vi "crio_9074_FPGA_Load_Cell_new.vi"() -> ()   [LabVIEW 2019]
uses:
  <vilib>/LabVIEW Targets/FPGA/cRIO/shared/nicrio_ModuleControls/nicrio_cRIO-9237_DataRatesRing.ctl
  <vilib>/LabVIEW Targets/FPGA/cRIO/shared/nicrio_ModuleControls/nicrio_cRIO-9237_ExcitationVoltageRing.ctl
  <vilib>/rvi/Emulation/niFpgaSctlEmulationGetInTimedLoop.vi
  <vilib>/rvi/Emulation/niFpgaProcessEmulError.vi
  <vilib>/rvi/eio/common/nirviEmuTemplatePropertySet_errors.vi
  <vilib>/rvi/eio/common/nirviEmuTemplateMethod_errors.vi
  <vilib>/rvi/Emulation/niFpgaGetClockAttributes.vi
  <vilib>/rvi/Emulation/niFpgaEmulationReportErrorSimple.vi
  <vilib>/rvi/Emulation/niFpgaCriticalErrorInLSC.vi
  <vilib>/eio/EIOPropertyNode/EIOPropertyNode.xnode
  <vilib>/eio/EIONode/EIONode.xnode
  <vilib>/rvi/eio/common/nirviEmuTemplatePropertyGet_errors.vi
  <vilib>/rvi/eio/common/nirviEmuTemplatePropertyGet_noerrors.vi
  <vilib>/rvi/eio/common/nirviEmuTemplatePropertySet_noerrors.vi
panel:
  in  "Loop Rate (uSec)":u32
  out "Mod1/AI0":fxp<+/-,24,-4>
  in  "Half-Bridge Enable":bool
  in  "Excitation Voltage":T1 items=["2.5 Volts", "3.3 Volts", "5.0 Volts", "10.0 Volts", "External Excitation"]
  in  "Finite?":bool=TRUE
  in  "Samples per Channel":u32=1000
  in  "Shunt Cal Enable":bool
  in  "Stop Button":bool
  in  "Data Rate":T2=1 items=["50.000 kS/s (NI 9237)"=1, "25.000 kS/s (NI 9237)"=2, "16.667 kS/s (NI 9237)"=3, "12.500 kS/s (NI 9237)"=4, "10.000 kS/s (NI 9237)"=5, "8.333 kS/s (NI 9237)"=6, "7.143 kS/s (NI 9237)"=7, "6.250 kS/s (NI 9237)"=8, "5.556 kS/s (NI 9237)"=9, "5.000 kS/s (NI 9237)"=10, "4.545 kS/s (NI 9237)"=11, "4.167 kS/s (NI 9237)"=12, "3.846 kS/s (NI 9237)"=13, "3.571 kS/s (NI 9237)"=14, "3.333 kS/s (NI 9237)"=15, "3.125 kS/s (NI 9237)"=16, "2.941 kS/s (NI 9237)"=17, "2.778 kS/s (NI 9237)"=18, "2.632 kS/s (NI 9237)"=19, "2.500 kS/s (NI 9237)"=20, "2.381 kS/s (NI 9237)"=21, "2.273 kS/s (NI 9237)"=22, "2.174 kS/s (NI 9237)"=23, "2.083 kS/s (NI 9237)"=24, "2.000 kS/s (NI 9237)"=25, "1.923 kS/s (NI 9237)"=26, "1.852 kS/s (NI 9237)"=27, "1.786 kS/s (NI 9237)"=28, "1.724 kS/s (NI 9237)"=29, "1.667 kS/s (NI 9237)"=30, "1.613 kS/s (NI 9237)"=31]
  out "error out":errorcluster {"code" format="%.0x"}
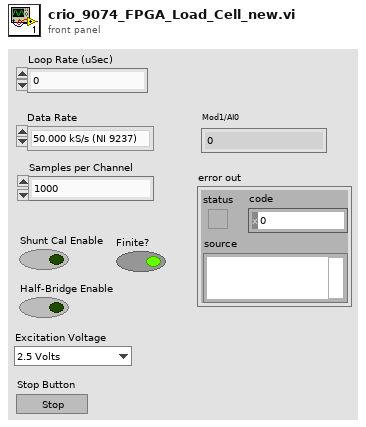
[diagram p1: front panel]
types:
  T1 = typedef "nicrio_cRIO-9237_ExcitationVoltageRing.ctl" = u8
  T2 = typedef "nicrio_cRIO-9237_DataRatesRing.ctl" = u8
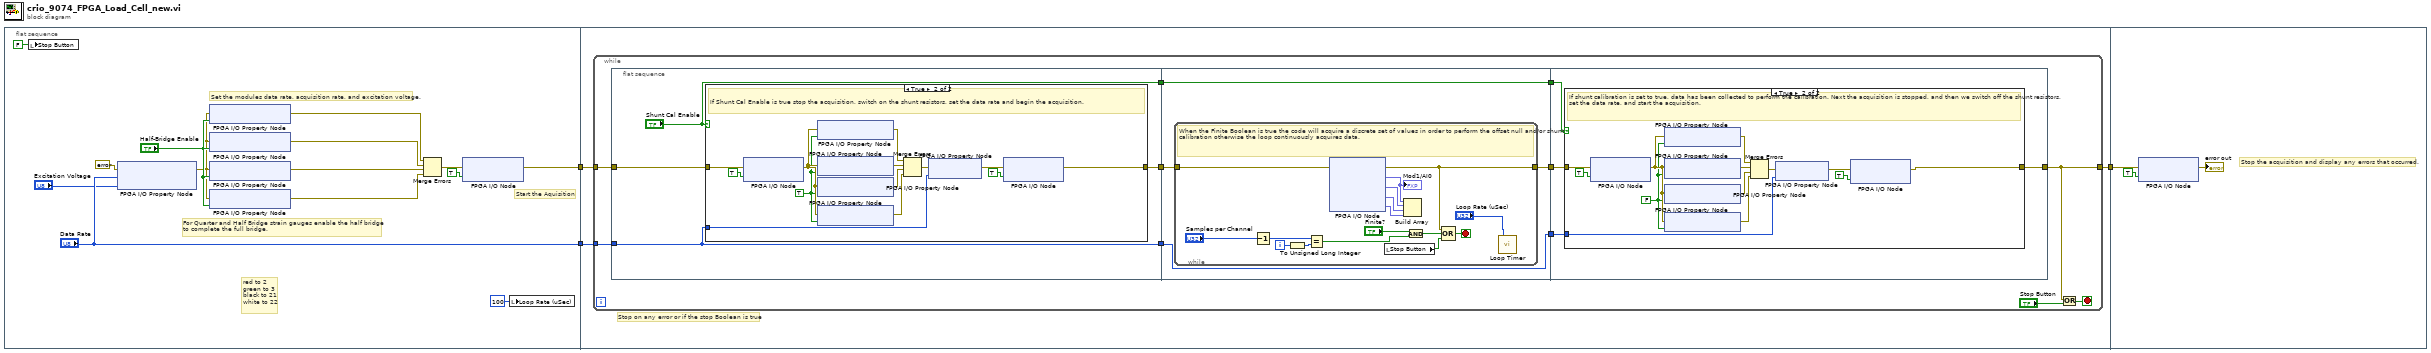
[diagram p0: block diagram]
diagram:
  n1 = flat-sequence {
    tunnel: [w16] -> w3
    tunnel: ["Data Rate"] -> w2
    tunnel: w3 -> [w20]
    tunnel: w2 -> [w19]
    tunnel: [w18] -> w1
    tunnel: w1 -> [w89]
    frame #0 {
      # "red to 2\ngreen to 3\nblack to 21\nwhite to 22"
      # "Start the Aquisition"
      # "For Quarter and Half Bridge strain gauges enable the half bridge \nto complete the full bridge."
      # "Set the modules data rate, acquisition rate, and excitation voltage."
      n2 = local write "Stop Button"(FALSE ("Stop Button")) -> ()
      n3 = xnode "FPGA I/O Property Node"("error in"=errorcluster {"status"=FALSE, "code"=0, "source"=""}, "Data Rate"="Data Rate", "Excitation Voltage"="Excitation Voltage") -> ("error out"=w7:errorcluster)  [unwired: 1 in, 1 out]
      n4 = xnode "FPGA I/O Property Node"("error in"=w7, "Half-Bridge Enable"="Half-Bridge Enable") -> ("error out"=w11:errorcluster)  [unwired: 1 in, 1 out]
      n5 = xnode "FPGA I/O Property Node"("error in"=w7, "Half-Bridge Enable"="Half-Bridge Enable") -> ("error out"=w10:errorcluster)  [unwired: 1 in, 1 out]
      n6 = xnode "FPGA I/O Property Node"("error in"=w7, "Half-Bridge Enable"="Half-Bridge Enable") -> ("error out"=w9:errorcluster)  [unwired: 1 in, 1 out]
      n7 = xnode "FPGA I/O Property Node"("error in"=w7, "Half-Bridge Enable"="Half-Bridge Enable") -> ("error out"=w8:errorcluster)  [unwired: 1 in, 1 out]
      n8 = Merge Errors(w11, w10, w9, w8) -> (w6:errorcluster)
      n9 = xnode "FPGA I/O Node"("error in"=w6, "Mod6/Start"=TRUE ("Mod1/Stop")) -> ("error out"=w16:errorcluster)  [unwired: 1 in, 1 out]
      n10 = local write "Loop Rate (uSec)"(u32 100 ("Loop Rate (uSec)")) -> ()
    }
    frame #1 {
      # "Stop on any error or if the stop Boolean is true"
      n11 = while {
        tunnel: w20 -> [w31]
        tunnel: [w28] -> w18
        tunnel: w19 -> [w25]
        stop <- w29 stop-if-true
        n12 = flat-sequence {
          tunnel: [w34] -> w26
          tunnel: [w33] -> w23
          tunnel: ["Shunt Cal Enable"] -> w22
          tunnel: w25 -> [w33]
          tunnel: w31 -> [w35]
          tunnel: [w52] -> w30
          tunnel: w26 -> [w53]
          tunnel: [w51] -> w24
          tunnel: w23 -> [w51]
          tunnel: w22 -> [w50]
          tunnel: [w50] -> w21
          tunnel: [w72] -> w28
          tunnel: w30 -> [w73]
          tunnel: w24 -> [w70]
          tunnel: w21 -> [w71]
          frame #0 {
            n13 = case shown="True" "Shunt Cal Enable" {
              tunnel: w35 -> [w36 w46]
              tunnel: [w36 w44] -> w34
              tunnel: w33 -> [_ w41]
              frame False {
              }
              frame True {
                w39 = TRUE ("Shunt Cal Enable")
                # "If Shunt Cal Enable is true stop the acquisition, switch on the shunt resistors, set the data rate and begin the acquisition."
                n14 = xnode "FPGA I/O Node"("error in"=w46, "Mod6/Stop"=TRUE ("Mod1/Stop")) -> ("error out"=w45:errorcluster)  [unwired: 1 in, 1 out]
                n15 = xnode "FPGA I/O Property Node"("error in"=w45, "Shunt Cal Enable"=w39) -> ("error out"=w49:errorcluster)  [unwired: 1 in, 1 out]
                n16 = xnode "FPGA I/O Property Node"("error in"=w45, "Shunt Cal Enable"=w39) -> ("error out"=w37:errorcluster)  [unwired: 1 in, 1 out]
                n17 = xnode "FPGA I/O Property Node"("error in"=w45, "Shunt Cal Enable"=w39) -> ("error out"=w48:errorcluster)  [unwired: 1 in, 1 out]
                n18 = xnode "FPGA I/O Property Node"("error in"=w45, "Shunt Cal Enable"=w39) -> ("error out"=w47:errorcluster)  [unwired: 1 in, 1 out]
                n19 = Merge Errors(w49, w37, w48, w47) -> (w42:errorcluster)
                n20 = xnode "FPGA I/O Property Node"("error in"=w42, "Data Rate"=w41) -> ("error out"=w43:errorcluster)  [unwired: 1 in, 1 out]
                n21 = xnode "FPGA I/O Node"("error in"=w43, "Mod6/Start"=TRUE ("Mod1/Start")) -> ("error out"=w44:errorcluster)  [unwired: 1 in, 1 out]
              }
            }
          }
          frame #1 {
            n22 = while {
              tunnel: w53 -> [w55]
              tunnel: [w59] -> w52
              i -> [w63]
              stop <- w56 stop-if-true
              # "When the Finite Boolean is true the code will acquire a discrete set of values in order to perform the offset null and/or shunt calibration otherwise the loop continuously acquires data."
              n23 = Decrement(x="Samples per Channel") -> (x-1=w65:u32)
              n24 = To Unsigned Long Integer(number=w63) -> (unsigned 32bit integer=w64:u32)
              n25 = Equal?(x=w65, y=w64) -> (x = y?=w60:bool)
              n26 = xnode "FPGA I/O Node"("error in"=w55) -> ("error out"=w59:errorcluster, "Mod6/AI0"=w69:fxp<+/-,24,-4>, "Mod6/AI1"=w68:fxp<+/-,24,-4>, "Mod6/AI2"=w66:fxp<+/-,24,-4>, "Mod6/AI3"=w67:fxp<+/-,24,-4>)  [unwired: 4 in, 4 out]
              "Mod1/AI0" <- w69
              n27 = local read "Stop Button"() -> (w57:bool)
              n28 = Build Array(w69, w68, w66, w67) -> ()  [unwired: 1 out]
              n29 = And(x="Finite?", y=w60) -> (x .and. y?=w58:bool)
              n30 = Compound Arithmetic op=OR(w59, w58, w57) -> (w56:bool)
              n31 = call "Loop Timer"("Count(uSec)"="Loop Rate (uSec)") -> ()  [unwired: 1 out]
            }
          }
          frame #2 {
            n32 = case shown="True" w71 {
              tunnel: w73 -> [w74 w83]
              tunnel: [w74 w81] -> w72
              tunnel: w70 -> [_ w78]
              frame False {
              }
              frame True {
                w77 = FALSE ("Shunt Cal Enable")
                # "If shunt calibration is set to true, data has been collected to perform the calibration. Next the acquisition is stopped, and then we switch off the shunt resistors, set the data rate, and start the acquisition."
                n33 = xnode "FPGA I/O Node"("error in"=w83, "Mod6/Stop"=TRUE ("Mod1/Stop")) -> ("error out"=w82:errorcluster)  [unwired: 1 in, 1 out]
                n34 = xnode "FPGA I/O Property Node"("error in"=w82, "Shunt Cal Enable"=w77) -> ("error out"=w87:errorcluster)  [unwired: 1 in, 1 out]
                n35 = xnode "FPGA I/O Property Node"("error in"=w82, "Shunt Cal Enable"=w77) -> ("error out"=w86:errorcluster)  [unwired: 1 in, 1 out]
                n36 = xnode "FPGA I/O Property Node"("error in"=w82, "Shunt Cal Enable"=w77) -> ("error out"=w85:errorcluster)  [unwired: 1 in, 1 out]
                n37 = xnode "FPGA I/O Property Node"("error in"=w82, "Shunt Cal Enable"=w77) -> ("error out"=w84:errorcluster)  [unwired: 1 in, 1 out]
                n38 = Merge Errors(w87, w86, w85, w84) -> (w79:errorcluster)
                n39 = xnode "FPGA I/O Property Node"("error in"=w79, "Data Rate"=w78) -> ("error out"=w80:errorcluster)  [unwired: 1 in, 1 out]
                n40 = xnode "FPGA I/O Node"("error in"=w80, "Mod6/Start"=TRUE ("Mod1/Start")) -> ("error out"=w81:errorcluster)  [unwired: 1 in, 1 out]
              }
            }
          }
        }
        n41 = Or(x=w28, y="Stop Button") -> (x .or. y?=w29:bool)
      }
    }
    frame #2 {
      # "Stop the acquisition and display any errors that occurred."
      n42 = xnode "FPGA I/O Node"("error in"=w89, "Mod6/Stop"=TRUE ("Mod1/Stop")) -> ("error out"=→"error out":errorcluster)  [unwired: 1 in, 1 out]
    }
  }
